vi "waypoint.vi"(6 "color(black)":u32(colorbox), 9 "picture":picture, 10 "waypointy":dbl, 11 "waypointx":dbl) -> (2 "new picture":picture)   [LabVIEW 2016]
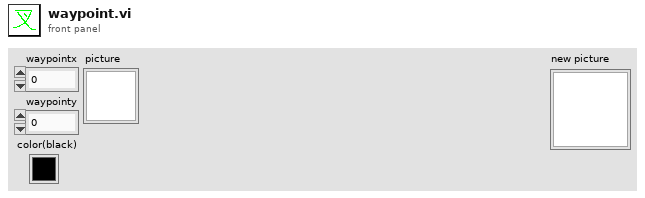
[diagram p1: front panel]
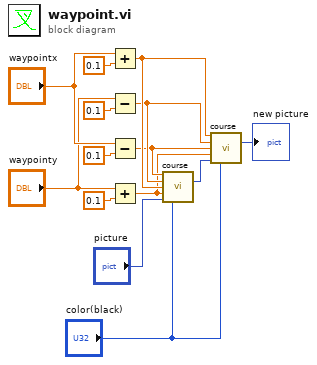
[diagram p0: block diagram]
diagram:
  n1 = Add(x="waypointx", y=0.1) -> (x+y=w4:dbl)
  n2 = Subtract(x="waypointy", y=0.1) -> (x-y=w3:dbl)
  n3 = Subtract(x="waypointx", y=0.1) -> (x-y=w2:dbl)
  n4 = Add(x="waypointy", y=0.1) -> (x+y=w1:dbl)
  n5 = call "course.vi"("x1"=w2, "y 1"=w3, "x2"=w4, "y 2"=w1, "picture"="picture", "color(black)"="color(black)") -> ("new picture"=w5:picture)  [unwired: 9 in]
  n6 = call "course.vi"("x1"=w4, "y 1"=w3, "x2"=w2, "y 2"=w1, "picture"=w5, "color(black)"="color(black)") -> ("new picture"=→"new picture":picture)  [unwired: 9 in]
